vi "initialize AI phase task.vi"(8 "error in (no error)":errorcluster, 11 "NI in":refnum<class "NI.lvclass">) -> (0 "error out":errorcluster, 3 "NI out":refnum<class "NI.lvclass">)   [LabVIEW 2021, in "NI.lvlib" / "NI.lvclass"]
uses:
  NI.lvclass
  NI.lvclass/NI.ctl
  <vilib>/DAQmx/create/channels.llb/DAQmx Create Channel (AI-Voltage-Basic).vi
  <vilib>/DAQmx/configure/timing.llb/DAQmx Timing (Sample Clock).vi
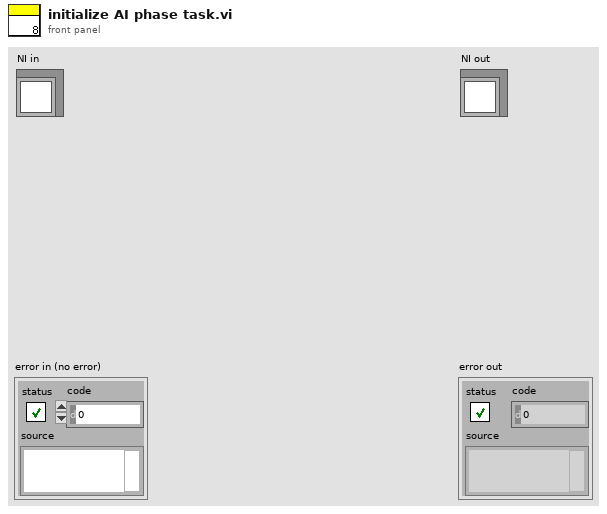
[diagram p1: front panel]
types:
  T1 = typedef "NI.lvlib/NI.lvclass/Channel Connection.ctl" = cluster{"Physical Channel":tag, "Terminal":tag, "StartTrigger":tag, "ClockSource":tag}
  T2 = cluster{"fast clock params":cluster{"fast clock rate":dbl, "off time after trigger":dbl, "cam line read time":dbl, "protect ticks #":dbl}, "AO1 laser Connection":T1, "AO2 zy Connection":T1, "AO3 z Connection (deprecated)":T1, "CO1 mainTrig Connection":T1, "CO2 fastClock Connection":T1, "AI phase Connection":T1}
  T3 = typedef "NI.lvlib/NI.lvclass/NI task parameters.ctl" = cluster{"exposure time":dbl, "camera H":dbl, "y line #":dbl, "flyback line #":dbl, "y pixel size":dbl, "z scan #":dbl, "z step size":dbl, "z offset":dbl, "laser all on?":bool, "laser option":bool[]}
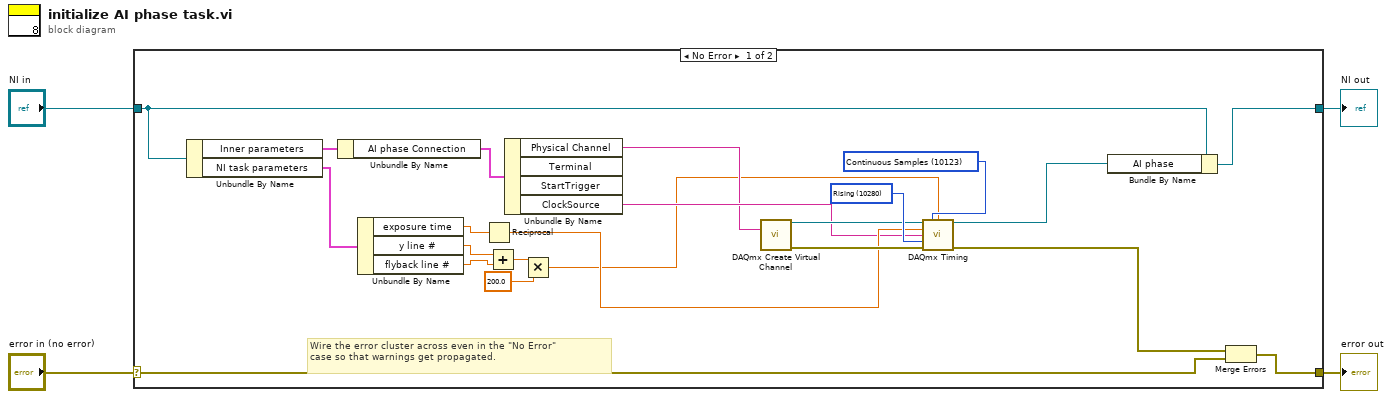
[diagram p0: block diagram]
diagram:
  n1 = case shown="No Error" "error in (no error)" {
    selector: "error in (no error)" -> [w7 w28]
    tunnel: [w6 w28] -> w3
    tunnel: [w14 w27] -> w1
    tunnel: "NI in" -> [w15 w27]
    frame No Error {
      w23 = 10280 items=["Rising"=10280, "Falling"=10171] ("active edge")
      w20 = 10123 items=["Finite Samples"=10178, "Continuous Samples"=10123, "Hardware Timed Single Point"=12522] ("sample mode")
      # "Wire the error cluster across even in the \"No Error\"\ncase so that warnings get propagated."
      n2 = Unbundle By Name(w15) -> ("Inner parameters"=w26:T2, "NI task parameters"=w24:T3)
      n3 = Unbundle By Name(w26) -> ("AI phase Connection"=w25:T1)
      n4 = Unbundle By Name(w24) -> ("exposure time"=w19:dbl, "y line #"=w12:dbl, "flyback line #"=w11:dbl)
      n5 = Reciprocal(x=w19) -> (1/x=w18:dbl)
      n6 = Add(x=w12, y=w11) -> (x+y=w10:dbl)
      n7 = Unbundle By Name(w25) -> ("Physical Channel"=w16:tag, "ClockSource"=w17:tag)  [unwired: 2 out]
      n8 = Multiply(x=w10, y=200.0) -> (x*y=w8:dbl)
      n9 = call-poly <vilib>:"DAQmx Create Virtual Channel.vi"("physical channels"=w16) -> ("task out"=w22:refnum<k21>, "error out"=w21:errorcluster)  [unwired: 13 in]
      n10 = call-poly <vilib>:"DAQmx Timing.vi"("task/channels in"=w22, "sample mode"=w20, "samples per channel"=w8, "rate"=w18, "source"=w17, "active edge"=w23, "error in"=w21) -> ("task out"=w13:refnum<k21>, "error out"=w5:errorcluster)  [unwired: 7 in]
      n11 = Bundle By Name(cluster=w15, "AI phase"=w13) -> (w14:refnum<class "NI.lvclass">)
      n12 = Merge Errors(w5, w7) -> (w6:errorcluster)
    }
    frame Error {
    }
  }
  "error out" <- w3
  "NI out" <- w1
